vi "Read Camera.vi"(8 "error in (no error)":errorcluster, 11 "AMG8833 8x8 Camera in":refnum<class "AMG8833 8x8 Camera.lvclass">) -> (0 "error out":errorcluster, 2 "Camera Output":dbl[][](array[numeric]), 3 "AMG8833 8x8 Camera out":refnum<class "AMG8833 8x8 Camera.lvclass">)   [LabVIEW 2020, in "CTI-Peripheral.lvlib" / "AMG8833 8x8 Camera.lvclass"]
uses:
  AMG8833 8x8 Camera.lvclass
  AMG8833 8x8 Camera.lvclass/AMG8833 8x8 Camera.ctl
  CTI/I2C Connection/I2C Connection.lvclass/I2C Connection.ctl
  CTI/Session/I2C Write Data.vi
  CTI/Session/I2C Read Data.vi
  CTI/I2C Connection/I2C Connection.lvclass
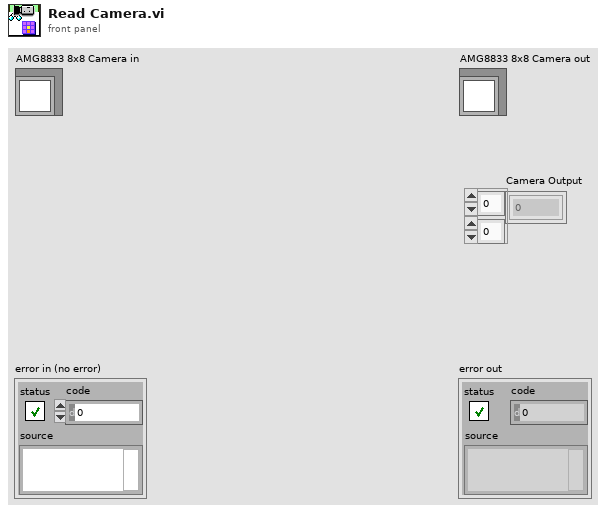
[diagram p1: front panel]
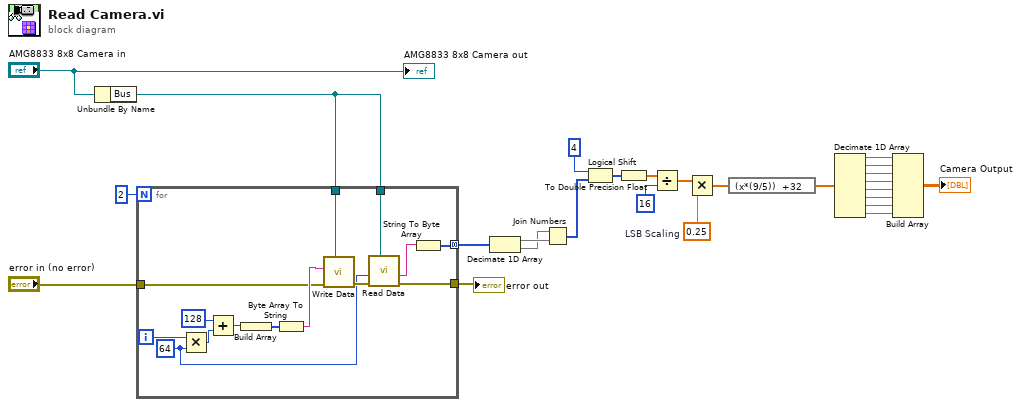
[diagram p0: block diagram]
diagram:
  w4 = 0.25  # LSB Scaling
  n1 = Unbundle By Name("AMG8833 8x8 Camera in") -> ("Bus"=w23:refnum<class "I2C Connection.lvclass">)
  n2 = for {
    N: 2 -> [_]
    tunnel: [w39] -> w3 mode=concatenating
    tunnel: "error in (no error)" -> [w31]
    tunnel: [w29] -> w1
    tunnel: w23 -> [w28]
    tunnel: w23 -> [w27]
    i -> [w37]
    w32 = u8 64 ("Read Len")
    n3 = Multiply(x=w37, y=w32) -> (x*y=w35:i32)
    n4 = Add(x=u8 128 ("Address"), y=w35) -> (x+y=w36:i32)
    n5 = Build Array(w36) -> (w40:i32[])
    n6 = Byte Array To String(unsigned byte array=w40) -> (string=w34:string)
    n7 = call "Write Data.vi"("I2C Connection"=w28, "error in (no error)"=w31, "Data"=w34) -> ("error out"=w33:errorcluster)  [unwired: 8 in]
    n8 = call "Read Data.vi"("I2C Connection"=w27, "error in (no error)"=w33, "Len"=w32) -> ("error out"=w29:errorcluster, "Data"=w30:string)  [unwired: 7 in]
    n9 = String To Byte Array(string=w30) -> (unsigned byte array=w39:u8[])
  }
  "error out" <- w1
  n10 = Decimate 1D Array(w3) -> (w22:u8[], w21:u8[])
  n11 = Join Numbers(hi=w21, lo=w22) -> ((hi.lo)=w8:u16[])
  n12 = Logical Shift(y=i16 4, x=w8) -> (x << y=w11:u16[])
  n13 = To Double Precision Float(number=w11) -> (double precision float=w10:dbl[])
  n14 = Divide(x=w10, y=i16 16) -> (x/y=w7:dbl[])
  n15 = Multiply(x=w7, y=w4) -> (x*y=w5:dbl[])
  n16 = expression code="(x*(9/5))  +32"(w5) -> (w6:dbl[])
  n17 = Decimate 1D Array(w6) -> (w13:dbl[], w14:dbl[], w15:dbl[], w16:dbl[], w17:dbl[], w18:dbl[], w19:dbl[], w20:dbl[])
  n18 = Build Array(w13, w14, w15, w16, w17, w18, w19, w20) -> (→"Camera Output":dbl[][])
  "AMG8833 8x8 Camera out" <- "AMG8833 8x8 Camera in"
